vi "Teleop.vi"(10 "Match Info":T1={"Autonomous Elapsed Seconds"=0.0, "TeleOp Elapsed Seconds"=0.0, "Disabled Elapsed Seconds"=0.0, "Visited Autonomous"=FALSE, "Visited TeleOp"=FALSE, "Visited Disabled"=FALSE, "Autonomous Settings"={"Autonomous Style"=enum."Independent", "VI Refnum"=refnum}}, 11 "Call Context":T2) -> ()   [LabVIEW 2019]
doc: "This VI is called for each enabled TeleOp packet received from the DS. It is typically used to read from joysticks and other inputs and update I/O or setpoints for timed control loops. It should complete and return within 20 milliseconds or risk missing DS packets."
uses:
  <vilib>/Rock Robotics/WPI/DriverStation/WPI_DriverStationDerivedRobotMode.ctl
  <vilib>/Rock Robotics/WPI/DriverStation/WPI_DriverStationMatch Info.ctl
  Framework/Robot Global Data.vi
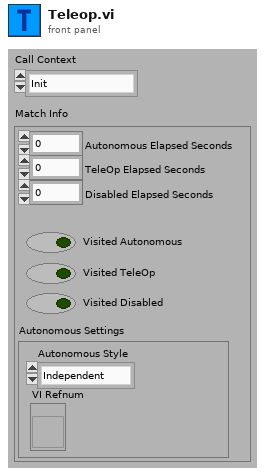
[diagram p1: front panel]
types:
  T1 = typedef "WPI_DriverStationMatch Info.ctl" = cluster{"Autonomous Elapsed Seconds":dbl, "TeleOp Elapsed Seconds":dbl, "Disabled Elapsed Seconds":dbl, "Visited Autonomous":bool, "Visited TeleOp":bool, "Visited Disabled":bool, "Autonomous Settings":cluster{"Autonomous Style":enum16{"Iterative", "Independent"}, "VI Refnum":refnum<vi>}}
  T2 = typedef "WPI_DriverStationDerivedRobotMode.ctl" = enum16{"Init", "Execute", "Stop"}
  T3 = typedef "Command Status Info.ctl" = cluster{"Name":string, "Status":T4, "notifier out":T5}
  T4 = typedef "Completion Status.ctl" = enum16{"Successful", "Aborted", "Incomplete"}
  T5 = typedef "Completion Notifier.ctl" = refnum<notifier>
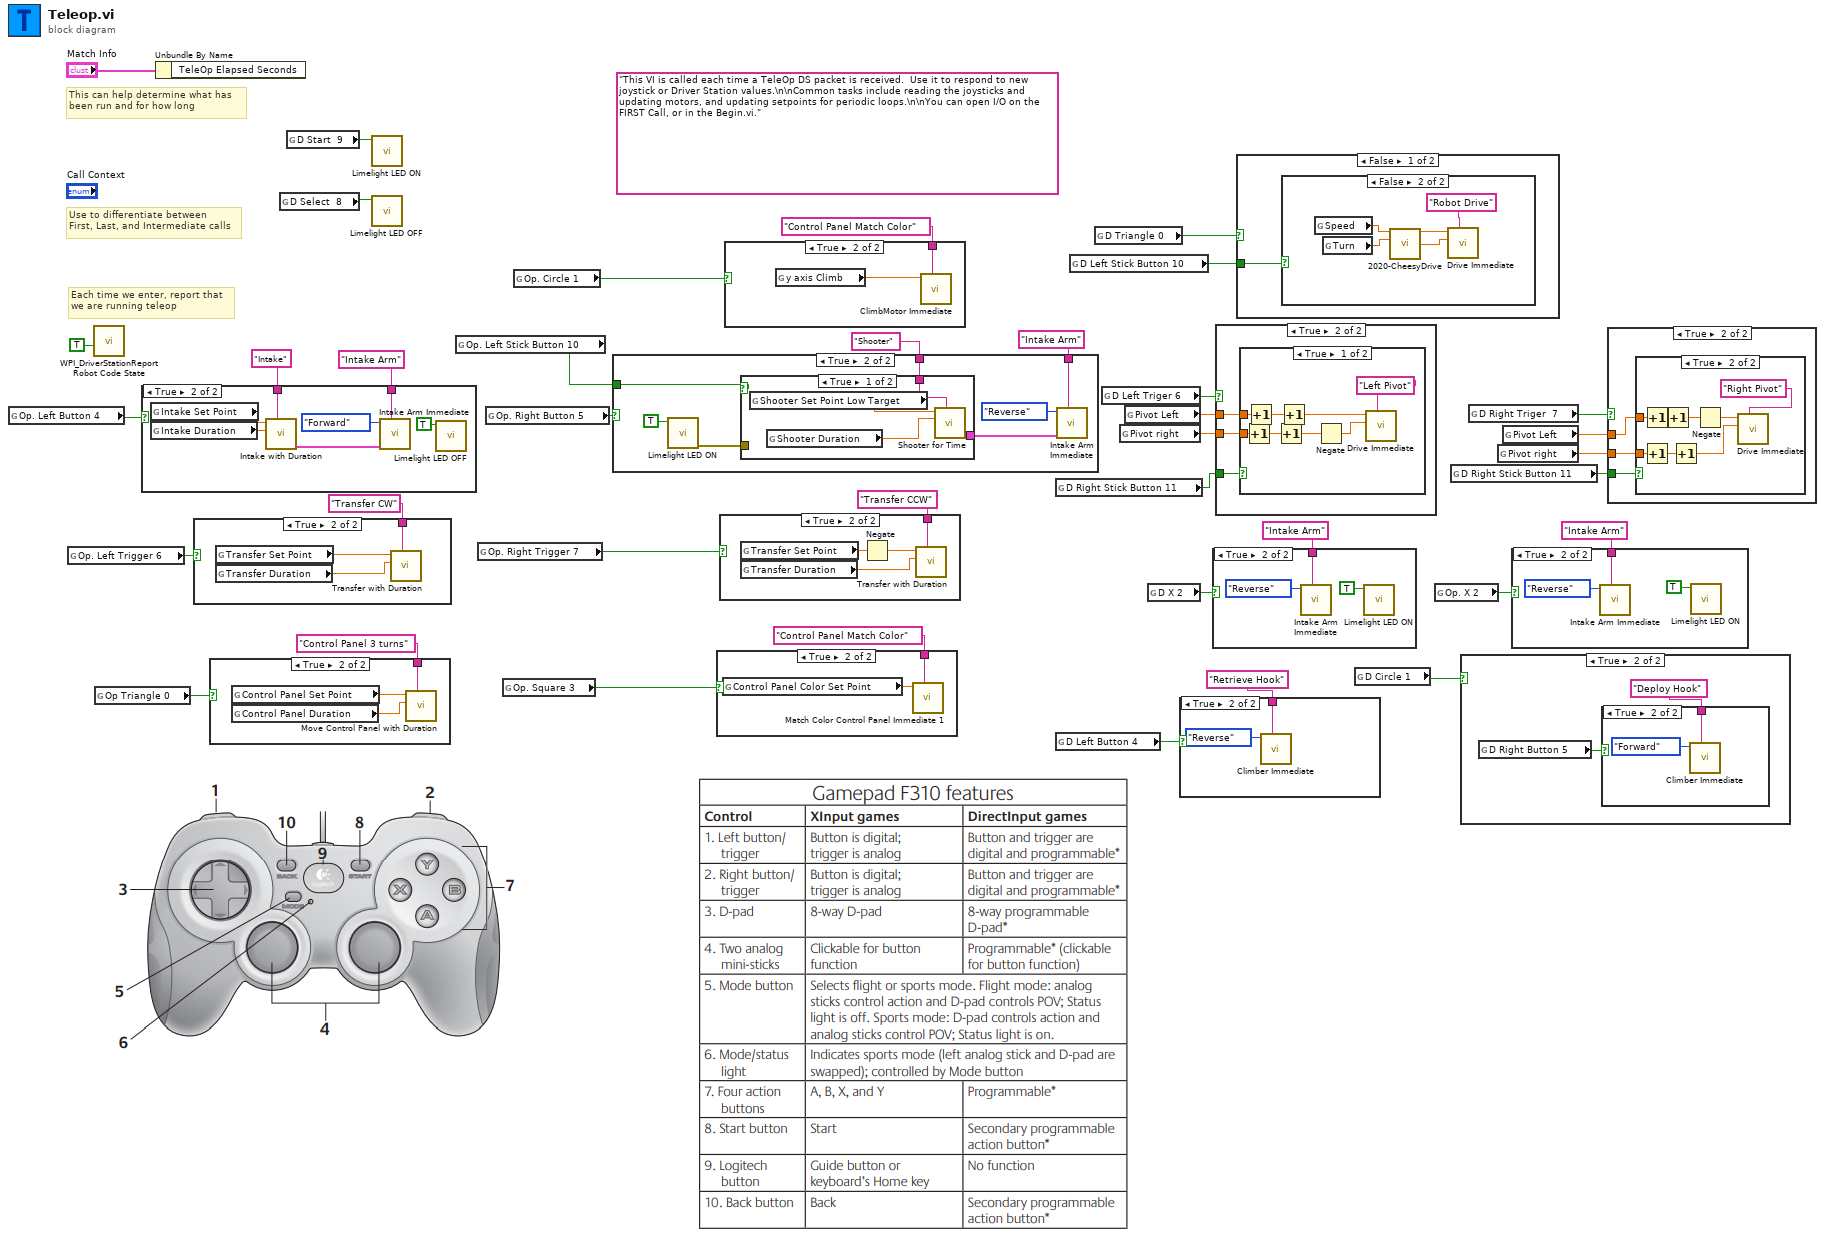
[diagram p0: block diagram]
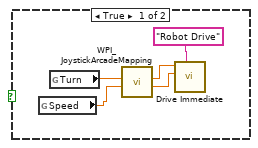
[diagram p7: hidden frame]
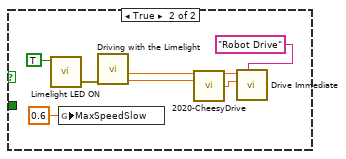
[diagram p8: hidden frame]
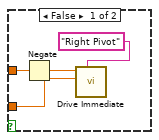
[diagram p13: hidden frame]
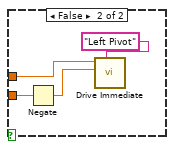
[diagram p15: hidden frame]
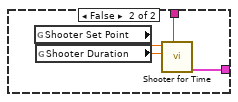
[diagram p19: hidden frame]
diagram:
  (unwired) "This VI is called each time a TeleOp DS packet is received.  Use it to respond to new joystick or Driver Station values.\n\nCommon tasks include reading the joysticks and updating motors, and updating setpoints for periodic loops.\n\nYou can open I/O on the FIRST Call, or in the Begin.vi."
  # "Each time we enter, report that\nwe are running teleop"
  # "Use to differentiate between\nFirst, Last, and Intermediate calls"
  # "This can help determine what has\nbeen run and for how long"
  n1 = global read "Robot Global Data.vi" "Op. Left Button 4"() -> (w36:bool)
  n2 = global read "Robot Global Data.vi" "Op. Left Trigger 6"() -> (w30:bool)
  n3 = call <vilib>:"WPI_DriverStationReport Robot Code State.vi"("TeleOp"=TRUE ("Autonomous")) -> ()  [unwired: 10 in, 1 out]
  n4 = global read "Robot Global Data.vi" "Op Triangle 0"() -> (w23:bool)
  n5 = case shown="True" w36 {
    tunnel: "Intake" ("refnum name") -> [_ w45]
    tunnel: "Intake Arm" ("refnum name") -> [_ w41]
    frame False {
    }
    frame True {
      n6 = global read "Robot Global Data.vi" "Intake Set Point"() -> (w44:dbl)
      n7 = global read "Robot Global Data.vi" "Intake Duration"() -> (w43:dbl)
      n8 = call "Intake with Duration.vi"("Description"=w45, "Duration (s)"=w43, "Setpoint"=w44) -> ("Command Info Out"=w40:T3)  [unwired: 8 in]
      n9 = call "Intake Arm Immediate.vi"("Description"=w41, "Command Info In"=w40, "Relay Value"=enum16{"Off", "On", "Forward", "Reverse"}."Forward") -> ()  [unwired: 8 in, 1 out]
      n10 = call "Limelight LED OFF.vi"("D Select  8"=TRUE) -> ()  [unwired: 11 in]
    }
  }
  n11 = Unbundle By Name("Match Info") -> ()  [unwired: 1 out]
  n12 = case shown="True" w30 {
    tunnel: "Transfer CW" ("refnum name") -> [_ w48]
    frame False {
    }
    frame True {
      n13 = global read "Robot Global Data.vi" "Transfer Set Point"() -> (w47:dbl)
      n14 = global read "Robot Global Data.vi" "Transfer Duration"() -> (w46:dbl)
      n15 = call "Transfer with Duration.vi"("Description"=w48, "Duration (s)"=w46, "Setpoint"=w47) -> ()  [unwired: 8 in, 1 out]
    }
  }
  n16 = case shown="True" w23 {
    tunnel: "Control Panel 3 turns" ("refnum name") -> [_ w51]
    frame False {
    }
    frame True {
      n17 = global read "Robot Global Data.vi" "Control Panel Set Point"() -> (w50:dbl)
      n18 = global read "Robot Global Data.vi" "Control Panel Duration"() -> (w49:dbl)
      n19 = call "Move Control Panel with Duration.vi"("Description"=w51, "Duration (s)"=w49, "Setpoint"=w50) -> ()  [unwired: 8 in, 1 out]
    }
  }
  n20 = global read "Robot Global Data.vi" "D Select  8"() -> (w4:bool)
  n21 = global read "Robot Global Data.vi" "D Start  9"() -> (w5:bool)
  n22 = call "Limelight LED ON.vi"("D Start  9"=w5) -> ()  [unwired: 10 in, 1 out]
  n23 = call "Limelight LED OFF.vi"("D Select  8"=w4) -> ()  [unwired: 11 in]
  n24 = global read "Robot Global Data.vi" "Op. Left Stick Button 10"() -> (w6:bool)
  n25 = global read "Robot Global Data.vi" "Op. Right Trigger 7"() -> (w31:bool)
  n26 = global read "Robot Global Data.vi" "Op. Right Button 5"() -> (w32:bool)
  n27 = global read "Robot Global Data.vi" "Op. Square 3"() -> (w20:bool)
  n28 = global read "Robot Global Data.vi" "Op. Circle 1"() -> (w8:bool)
  n29 = case shown="True" w32 {
    tunnel: "Shooter" ("refnum name") -> [_ w58]
    tunnel: "Intake Arm" ("refnum name") -> [_ w56]
    tunnel: w6 -> [_ w54]
    frame False {
    }
    frame True {
      n30 = call "Limelight LED ON.vi"("D Start  9"=TRUE) -> ("error out"=w52:errorcluster)  [unwired: 10 in]
      n31 = case shown="True" w54 {
        tunnel: w58 -> [w62 w66]
        tunnel: [w59 w63] -> w55
        tunnel: w52 -> [_ _]
        frame True {
          n32 = global read "Robot Global Data.vi" "Shooter Set Point Low Target"() -> (w61:dbl)
          n33 = global read "Robot Global Data.vi" "Shooter Duration"() -> (w60:dbl)
          n34 = call "Shooter for Time.vi"("Description"=w62, "Duration (s)"=w60, "Setpoint"=w61) -> ("Command Info Out"=w59:T3)  [unwired: 8 in]
        }
        frame False {
          n35 = global read "Robot Global Data.vi" "Shooter Set Point"() -> (w65:dbl)
          n36 = global read "Robot Global Data.vi" "Shooter Duration"() -> (w64:dbl)
          n37 = call "Shooter for Time.vi"("Description"=w66, "Duration (s)"=w64, "Setpoint"=w65) -> ("Command Info Out"=w63:T3)  [unwired: 8 in]
        }
      }
      n38 = call "Intake Arm Immediate.vi"("Description"=w56, "Command Info In"=w55, "Relay Value"=enum16{"Off", "On", "Forward", "Reverse"}."Reverse") -> ()  [unwired: 8 in, 1 out]
    }
  }
  n39 = case shown="True" w20 {
    tunnel: "Control Panel Match Color" ("refnum name") -> [_ w68]
    frame False {
    }
    frame True {
      n40 = global read "Robot Global Data.vi" "Control Panel Color Set Point"() -> (w67:dbl)
      n41 = call "Match Color Control Panel Immediate 1.vi"("Description"=w68, "Setpoint"=w67) -> ()  [unwired: 9 in, 1 out]
    }
  }
  n42 = case shown="True" w31 {
    tunnel: "Transfer CCW" ("refnum name") -> [_ w72]
    frame False {
    }
    frame True {
      n43 = global read "Robot Global Data.vi" "Transfer Set Point"() -> (w70:dbl)
      n44 = global read "Robot Global Data.vi" "Transfer Duration"() -> (w69:dbl)
      n45 = Negate(x=w70) -> (-x=w71:dbl)
      n46 = call "Transfer with Duration.vi"("Description"=w72, "Duration (s)"=w69, "Setpoint"=w71) -> ()  [unwired: 8 in, 1 out]
    }
  }
  n47 = case shown="True" w8 {
    tunnel: "Control Panel Match Color" ("refnum name") -> [_ w74]
    frame False {
    }
    frame True {
      n48 = global read "Robot Global Data.vi" "y axis Climb"() -> (w73:dbl)
      n49 = call "ClimbMotor Immediate.vi"("Description"=w74, "Setpoint"=w73) -> ()  [unwired: 9 in, 1 out]
    }
  }
  n50 = global read "Robot Global Data.vi" "D Right Stick Button 11"() -> (w1:bool)
  n51 = global read "Robot Global Data.vi" "D Left Button 4"() -> (w13:bool)
  n52 = global read "Robot Global Data.vi" "D Left Stick Button 10"() -> (w3:bool)
  n53 = global read "Robot Global Data.vi" "D Triangle 0"() -> (w14:bool)
  n54 = global read "Robot Global Data.vi" "D Left Triger 6"() -> (w28:bool)
  n55 = global read "Robot Global Data.vi" "Pivot right"() -> (w17:dbl)
  n56 = global read "Robot Global Data.vi" "Pivot Left"() -> (w18:dbl)
  n57 = global read "Robot Global Data.vi" "D X 2"() -> (w21:bool)
  n58 = case shown="True" w13 {
    tunnel: "Retrieve Hook" ("refnum name") -> [_ w75]
    frame False {
    }
    frame True {
      n59 = call "Climber Immediate.vi"("Description"=w75, "Value"=enum16{"Off", "On", "Forward", "Reverse"}."Reverse" ("Relay Value")) -> ()  [unwired: 9 in, 1 out]
    }
  }
  n60 = case shown="True" w21 {
    tunnel: "Intake Arm" ("refnum name") -> [_ w78]
    frame False {
    }
    frame True {
      n61 = call "Intake Arm Immediate.vi"("Description"=w78, "Relay Value"=enum16{"Off", "On", "Forward", "Reverse"}."Reverse") -> ()  [unwired: 9 in, 1 out]
      n62 = call "Limelight LED ON.vi"("D Start  9"=TRUE) -> ()  [unwired: 10 in, 1 out]
    }
  }
  n63 = case shown="True" w28 {
    tunnel: w18 -> [_ w82]
    tunnel: w17 -> [_ w81]
    tunnel: w1 -> [_ w80]
    frame False {
    }
    frame True {
      n64 = case shown="True" w80 {
        tunnel: w82 -> [w89 w93]
        tunnel: w81 -> [w88 w92]
        frame True {
          n65 = Increment(x=w88) -> (x+1=w84:dbl)
          n66 = Increment(x=w89) -> (x+1=w86:dbl)
          n67 = Increment(x=w84) -> (x+1=w83:dbl)
          n68 = Increment(x=w86) -> (x+1=w85:dbl)
          n69 = Negate(x=w83) -> (-x=w87:dbl)
          n70 = call "Drive Immediate.vi"("Description"="Left Pivot", "Right Setpoint"=w87, "Left Setpoint"=w85) -> ()  [unwired: 8 in, 1 out]
        }
        frame False {
          n71 = Negate(x=w92) -> (-x=w91:dbl)
          n72 = call "Drive Immediate.vi"("Description"="Left Pivot", "Right Setpoint"=w91, "Left Setpoint"=w93) -> ()  [unwired: 8 in, 1 out]
        }
      }
    }
  }
  n73 = case shown="False" w14 {
    tunnel: w3 -> [w95 _]
    frame False {
      n74 = case shown="False" w95 {
        frame True {
          n75 = global read "Robot Global Data.vi" "Speed"() -> (w98:dbl)
          n76 = global read "Robot Global Data.vi" "Turn"() -> (w99:dbl)
          n77 = call <vilib>:"WPI_JoystickArcadeMapping.vi"("Y axis value"=w98, "X axis value"=w99) -> ("Right Motor Value"=w96:dbl, "Left Motor Value"=w97:dbl)  [unwired: 8 in]
          n78 = call "Drive Immediate.vi"("Description"="Robot Drive", "Right Setpoint"=w96, "Left Setpoint"=w97) -> ()  [unwired: 8 in, 1 out]
        }
        frame False {
          n79 = global read "Robot Global Data.vi" "Speed"() -> (w102:dbl)
          n80 = global read "Robot Global Data.vi" "Turn"() -> (w103:dbl)
          n81 = call "2020-CheesyDrive.vi"("Throttle"=w102, "Wheel"=w103) -> ("Left PWM"=w104:dbl, "Right PWM"=w105:dbl)  [unwired: 12 in]
          n82 = call "Drive Immediate.vi"("Description"="Robot Drive", "Right Setpoint"=w105, "Left Setpoint"=w104) -> ()  [unwired: 8 in, 1 out]
        }
      }
    }
    frame True {
      n83 = call "Limelight LED ON.vi"("D Start  9"=TRUE) -> ("error out"=w108:errorcluster)  [unwired: 10 in]
      n84 = global write "Robot Global Data.vi" "MaxSpeedSlow"(0.6 ("MaxSpeedSlow")) -> ()
      n85 = call "Driving with the Limelight.vi"("error in (no error)"=w108) -> ("TurnCommand"=w109:dbl, "SpeedCommand"=w110:dbl)  [unwired: 8 in, 1 out]
      n86 = call "2020-CheesyDrive.vi"("Throttle"=w110, "Wheel"=w109) -> ("Left PWM"=w112:dbl, "Right PWM"=w113:dbl)  [unwired: 12 in]
      n87 = call "Drive Immediate.vi"("Description"="Robot Drive", "Right Setpoint"=w113, "Left Setpoint"=w112) -> ()  [unwired: 8 in, 1 out]
    }
  }
  n88 = global read "Robot Global Data.vi" "D Circle 1"() -> (w7:bool)
  n89 = global read "Robot Global Data.vi" "Op. X 2"() -> (w11:bool)
  n90 = global read "Robot Global Data.vi" "D Right Stick Button 11"() -> (w2:bool)
  n91 = case shown="True" w7 {
    frame False {
    }
    frame True {
      n92 = global read "Robot Global Data.vi" "D Right Button 5"() -> (w114:bool)
      n93 = case shown="True" w114 {
        tunnel: "Deploy Hook" ("refnum name") -> [_ w116]
        frame False {
        }
        frame True {
          n94 = call "Climber Immediate.vi"("Description"=w116, "Value"=enum16{"Off", "On", "Forward", "Reverse"}."Forward" ("Relay Value")) -> ()  [unwired: 9 in, 1 out]
        }
      }
    }
  }
  n95 = global read "Robot Global Data.vi" "D Right Triger  7"() -> (w27:bool)
  n96 = global read "Robot Global Data.vi" "Pivot right"() -> (w15:dbl)
  n97 = global read "Robot Global Data.vi" "Pivot Left"() -> (w16:dbl)
  n98 = case shown="True" w11 {
    tunnel: "Intake Arm" ("refnum name") -> [_ w119]
    frame False {
    }
    frame True {
      n99 = call "Intake Arm Immediate.vi"("Description"=w119, "Relay Value"=enum16{"Off", "On", "Forward", "Reverse"}."Reverse") -> ()  [unwired: 9 in, 1 out]
      n100 = call "Limelight LED ON.vi"("D Start  9"=TRUE) -> ()  [unwired: 10 in, 1 out]
    }
  }
  n101 = case shown="True" w27 {
    tunnel: w16 -> [_ w123]
    tunnel: w15 -> [_ w122]
    tunnel: w2 -> [_ w121]
    frame False {
    }
    frame True {
      n102 = case shown="True" w121 {
        tunnel: w123 -> [w126 w134]
        tunnel: w122 -> [w125 w133]
        frame False {
          n103 = Negate(x=w126) -> (-x=w124:dbl)
          n104 = call "Drive Immediate.vi"("Description"="Right Pivot", "Right Setpoint"=w125, "Left Setpoint"=w124) -> ()  [unwired: 8 in, 1 out]
        }
        frame True {
          n105 = Increment(x=w134) -> (x+1=w131:dbl)
          n106 = Increment(x=w133) -> (x+1=w129:dbl)
          n107 = Increment(x=w131) -> (x+1=w130:dbl)
          n108 = Increment(x=w129) -> (x+1=w128:dbl)
          n109 = Negate(x=w130) -> (-x=w132:dbl)
          n110 = call "Drive Immediate.vi"("Description"="Right Pivot", "Right Setpoint"=w128, "Left Setpoint"=w132) -> ()  [unwired: 8 in, 1 out]
        }
      }
    }
  }
